vi "PC Main.vi"() -> ()   [LabVIEW 2021]
panel:
  in  "stop":bool
  out "Loop Time [ms]":u32
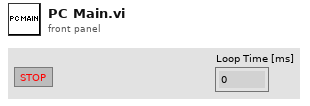
[diagram p1: front panel]
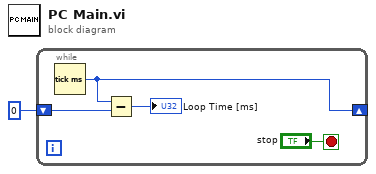
[diagram p0: block diagram]
diagram:
  n1 = while {
    shift-right: [w2] -> _
    shift-left: u32 0 ("millisecond timer value") -> [w3]
    stop <- "stop" stop-if-true
    n2 = Tick Count (ms)() -> (millisecond timer value=w2:u32)
    n3 = Subtract(x=w2, y=w3) -> (x-y=→"Loop Time [ms]":u32)
  }
